vi "process(Server).vi"(8 "error in (no error)":errorcluster, 10 "Sync":refnum<notifier>, 11 "Session in":refnum<class "Session.lvclass">) -> (0 "error out":errorcluster, 3 "Session out":refnum<class "Session.lvclass">)   [LabVIEW 2013]
uses:
  Session.lvclass
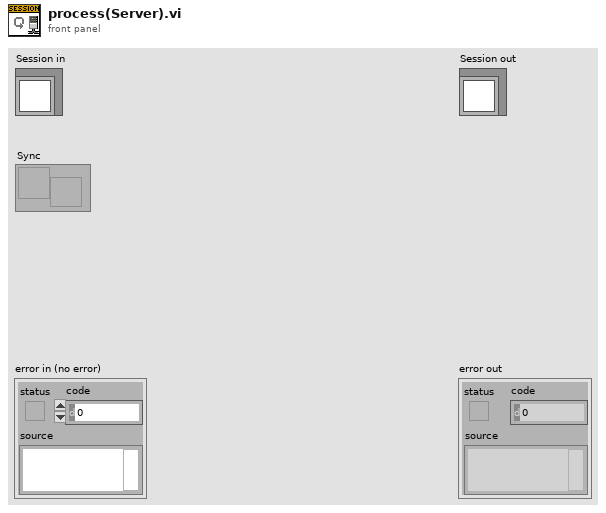
[diagram p1: front panel]
types:
  T1 = typedef "MQTT Base.lvlib/MQTT_Base.lvclass/Response -- cluster.ctl" = cluster{"Packet":refnum<class "ControlPacket.lvclass">, "Protocol Error":errorcluster, "disconnect session":bool, "[ACK]":refnum<notifier>[]}
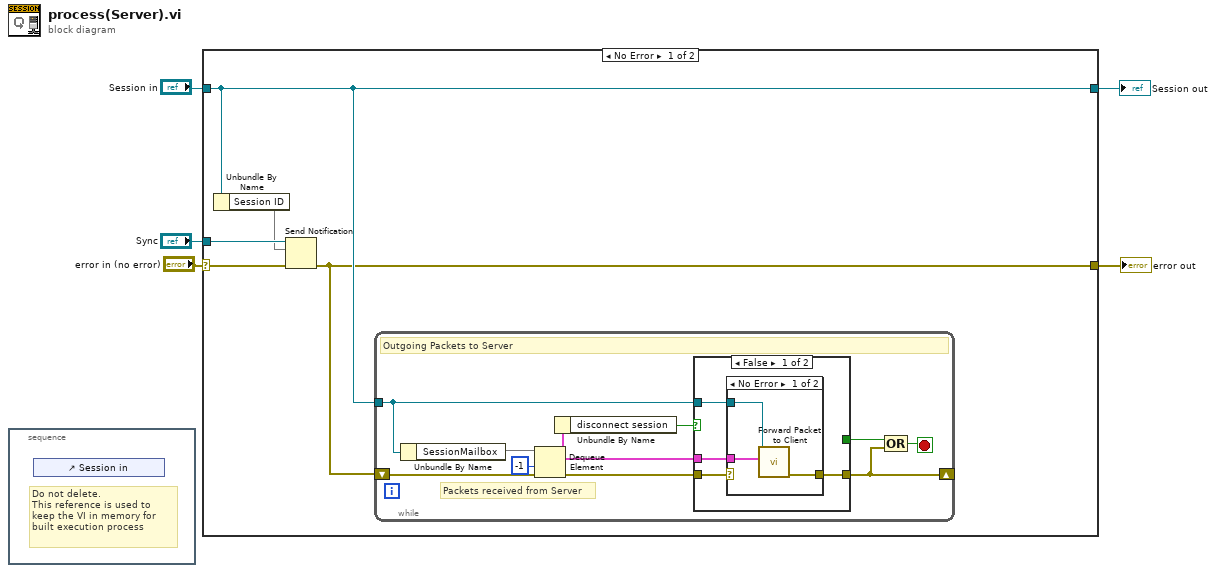
[diagram p0: block diagram]
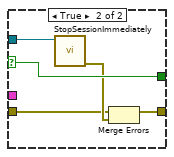
[diagram p3: hidden frame]
diagram:
  n1 = stacked-sequence {
    frame #0 {
      # "Do not delete.\nThis reference is used to keep the VI in memory for built execution process"
      n2 = control-ref of="Session in"() -> ()  [unwired: 1 out]
    }
  }
  n3 = case shown="No Error" "error in (no error)" {
    selector: "error in (no error)" -> [w9 w35]
    tunnel: [w6 w35] -> w3
    tunnel: [w7 w34] -> w2
    tunnel: "Session in" -> [w7 w34]
    tunnel: "Sync" -> [w10 _]
    frame No Error {
      n4 = Unbundle By Name(w7) -> ("Session ID"=w8)
      n5 = Send Notification(notification=w8, notifier=w10, error in (no error)=w9) -> (error out=w6:errorcluster)  [unwired: 1 out]
      n6 = while {
        tunnel: w7 -> [w16]
        shift-right: [w13] -> _
        shift-left: w6 -> [w17]
        stop <- w12 stop-if-true
        # "Packets received from Server"
        # "Outgoing Packets to Server"
        n7 = Unbundle By Name(w16) -> ("SessionMailbox"=w20)
        n8 = Dequeue Element(queue=w20, timeout in ms (-1)=-1, error in (no error)=w17) -> (element=w15:T1, error out=w18:errorcluster)  [unwired: 2 out]
        n9 = Unbundle By Name(w15) -> ("disconnect session"=w14:bool)
        n10 = case shown="False" w14 {
          selector: w14 -> [_ w33]
          tunnel: w18 -> [w24 w30]
          tunnel: [w23 w29] -> w13
          tunnel: w16 -> [w22 w32]
          tunnel: w15 -> [w21 _]
          tunnel: [_ w33] -> w11
          frame False {
            n11 = case shown="No Error" w24 {
              selector: w24 -> [_ w28]
              tunnel: w21 -> [w27 _]
              tunnel: [w26 w28] -> w23
              tunnel: w22 -> [w25 _]
              frame No Error {
                n12 = call "Forward Packet to Client.vi"("Response"=w27, "Session in"=w25) -> ("error out"=w26:errorcluster)  [unwired: 9 in]
              }
              frame Error {
              }
            }
          }
          frame True {
            n13 = call "StopSessionImmediately.vi"("Session in"=w32) -> ("error out"=w31:errorcluster)  [unwired: 9 in, 1 out]
            n14 = Merge Errors(w30, w31) -> (w29:errorcluster)
          }
        }
        n15 = Compound Arithmetic op=OR(w11, w13) -> (w12:bool)
      }
    }
    frame Error {
    }
  }
  "error out" <- w3
  "Session out" <- w2
